vi "In_S7F1.vi"(8 "error in (no error)":errorcluster, 11 "S7 Message Class in":refnum<class "S7 Message Class.lvclass">) -> (0 "error out":errorcluster, 1 "OK?":bool, 2 "S7F1":T1, 3 "S7 Message Class out":refnum<class "S7 Message Class.lvclass">)   [LabVIEW 2020, in "SECS Communication.lvlib" / "S7 Message Class.lvclass"]
uses:
  S7 Message Class.lvclass
  D:/Dropbox/SECS/SECS_GEM v1.0.6/Com/SECS Communication/SECS-II Class/SECS-II Class.lvclass
  S7F1.ctl
  SECS-II Class/SECS-II Class.lvclass/SECS-II Class.ctl
  SECS-II Class/Variant To Data_ASCII.vi
  SECS-II Class/Variant To Data_U4.vi
  SECS-II Class/SECS-II Class.lvclass
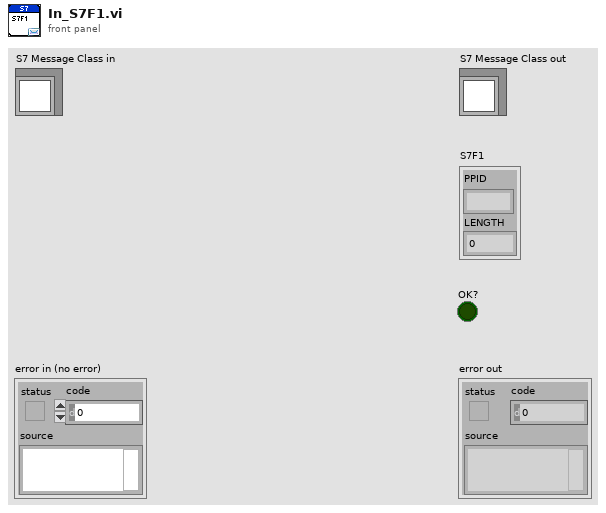
[diagram p1: front panel]
types:
  T1 = typedef "SECS Communication.lvlib/S7 Message Class.lvclass/S7F1.ctl" = cluster{"PPID":string, "LENGTH":u32}
  T2 = typedef "SECS Communication.lvlib/SECS-II Class.lvclass/Message Data.ctl" = cluster{"Index":i32, "Data Item Format":T3, "Format Code":T4, "Parent Index":i32, "Child Index":i32[], "Data":variant}
  T3 = typedef "SECS Communication.lvlib/SECS-II Class.lvclass/Data Item Format.ctl" = enum16{"Data Type", "Value"}
  T4 = typedef "SECS Communication.lvlib/SECS-II Class.lvclass/Format Code.ctl" = enum16{"L", "A", "B", "Boolean", "J", "I1", "I2", "I4", "I8", "U1", "U2", "U4", "U8", "F4", "F8", "Char"}
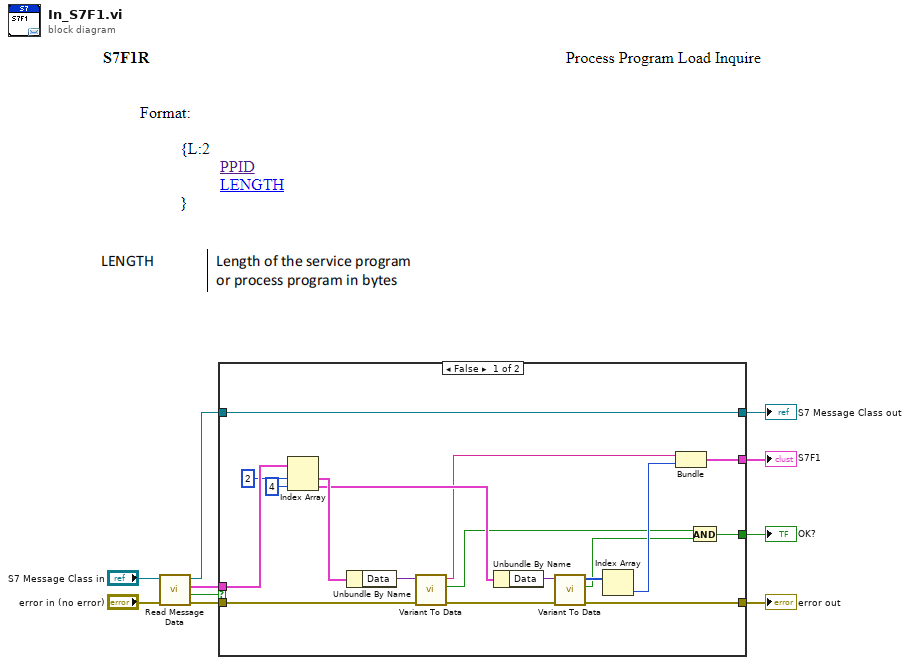
[diagram p0: block diagram]
diagram:
  n1 = call "Read Message Data.vi"("error in (no error)"="error in (no error)", "SECS-II Class in"="S7 Message Class in") -> ("error out"=w10:errorcluster, "Empty?"=w3:bool, "Message Data"=w9:T2[], "SECS-II Class out"=w2:refnum<class "S7 Message Class.lvclass">)  [unwired: 6 in]
  n2 = case shown="False" w3 {
    tunnel: w10 -> [w28 w30]
    tunnel: w9 -> [w27 _]
    tunnel: [w18 w30] -> w8
    tunnel: [w15 _] -> w5
    tunnel: [w12 _] -> w4
    tunnel: w2 -> [w11 w29]
    tunnel: [w11 w29] -> w1
    frame False {
      n3 = Index Array(array=w27, index #1=2 ("index"), index #2=4 ("index")) -> (element #1=w23:T2, element #2=w22:T2)
      n4 = Unbundle By Name(w23) -> ("Data"=w26:variant)
      n5 = call-poly "Variant To Data.vi"("error in (no error)"=w28, "Variant"=w26) -> ("error out"=w21:errorcluster, "OK?"=w13:bool, "Data"=w19:string)  [unwired: 7 in]
      n6 = Unbundle By Name(w22) -> ("Data"=w20:variant)
      n7 = call-poly "Variant To Data.vi"("error in (no error)"=w21, "Variant"=w20) -> ("error out"=w18:errorcluster, "OK?"=w14:bool, "Data"=w17:u32[])  [unwired: 7 in]
      n8 = Index Array(array=w17) -> (element=w16:u32)  [unwired: 1 in]
      n9 = Bundle("Data"=w19, "Data"=w16) -> (w15:cluster{"Data":string, "Data":u32})  [unwired: 1 in]
      n10 = And(x=w13, y=w14) -> (x .and. y?=w12:bool)
    }
    frame True {
    }
  }
  "error out" <- w8
  "S7 Message Class out" <- w1
  "S7F1" <- w5
  "OK?" <- w4
